vi "tx_top.vi"(0 "Modulation Parameters":T3 {"TX Parameters"."TX Sample Rate" items=["4M"]}) -> (9 "Transmitted IQ Graph":cluster{dbl[], dbl[]}(graph) caption="IQ Graph", 10 "Transmitted Magnitude":dbl[](graph), 11 "Transmitted Constellation Graph":T6(graph) caption="Constellation Graph", 13 "Transmitted Eye Diagram":cluster{"t0":dbl, "dt":dbl, "Y":dbl[]}[](graph) caption="Eye Diagram", 15 "Transmitted I":dbl[](graph), 16 "Transmitted Phase":dbl[](graph), 17 "Transmitted Q":dbl[](graph), 19 "Transmitted PSD":dbl[](graph), 20 "output IQ waveform":cluster{"t0":dbl, "dt":dbl, "Y":cdb[]}, 27 "error out":errorcluster)   [LabVIEW 2012]
uses:
  EE 497/LABS/SDR/control_type_defs.llb/tx_hw params.ctl
  EE 497/LABS/SDR/control_type_defs.llb/Queues.ctl
  gds_hw_config.lvlib
panel:
  in  "Queues in":T1
  in  "error in":errorcluster
  in  "STOP":bool
  out "Transmitting":bool
  out "Queues out":T1
  out "coerced gain (dB)":dbl format="%#_6f"
  out "coerced carrier frequency (Hz)":dbl format="%#_6p"
  out "data symbols":cdb[](array[numeric])=[0.0+0.0i, 0.7071067811865475+0.7071067811865475i, -0.7071067811865475-0.7071067811865475i, 0.7071067811865475-0.7071067811865475i, -0.7071067811865475-0.7071067811865475i, -0.7071067811865475+0.7071067811865475i, -0.7071067811865475+0.7071067811865475i, 0.7071067811865475-0.7071067811865475i, -0.7071067811865475+0.7071067811865475i, -0.7071067811865475-0.7071067811865475i, -0.7071067811865475+0.7071067811865475i, 0.7071067811865475-0.7071067811865475i, 0.7071067811865475+0.7071067811865475i, 0.7071067811865475-0.7071067811865475i, 0.7071067811865475-0.7071067811865475i, 0.7071067811865475+0.7071067811865475i, 0.7071067811865475+0.7071067811865475i, -0.7071067811865475+0.7071067811865475i, -0.7071067811865475+0.7071067811865475i, -0.7071067811865475-0.7071067811865475i, 0.7071067811865475-0.7071067811865475i, 0.7071067811865475+0.7071067811865475i, -0.7071067811865475-0.7071067811865475i, -0.7071067811865475-0.7071067811865475i, -0.7071067811865475-0.7071067811865475i, 0.7071067811865475-0.7071067811865475i, -0.7071067811865475+0.7071067811865475i, 0.7071067811865475-0.7071067811865475i, 0.7071067811865475+0.7071067811865475i, -0.7071067811865475+0.7071067811865475i, 0.7071067811865475-0.7071067811865475i, 0.7071067811865475-0.7071067811865475i, -0.7071067811865475+0.7071067811865475i, -0.7071067811865475-0.7071067811865475i, -0.7071067811865475-0.7071067811865475i, -0.7071067811865475-0.7071067811865475i, 0.7071067811865475+0.7071067811865475i, -0.7071067811865475+0.7071067811865475i, 0.7071067811865475-0.7071067811865475i, -0.7071067811865475+0.7071067811865475i, -0.7071067811865475+0.7071067811865475i, -0.7071067811865475+0.7071067811865475i, 0.7071067811865475-0.7071067811865475i, -0.7071067811865475+0.7071067811865475i, 0.7071067811865475-0.7071067811865475i, -0.7071067811865475+0.7071067811865475i, 0.7071067811865475+0.7071067811865475i, 0.7071067811865475+0.7071067811865475i, 0.7071067811865475+0.7071067811865475i, -0.7071067811865475-0.7071067811865475i, 0.7071067811865475+0.7071067811865475i, 0.7071067811865475-0.7071067811865475i, -0.7071067811865475+0.7071067811865475i, 0.7071067811865475-0.7071067811865475i, 0.7071067811865475-0.7071067811865475i, 0.7071067811865475+0.7071067811865475i, 0.7071067811865475-0.7071067811865475i, -0.7071067811865475+0.7071067811865475i, -0.7071067811865475+0.7071067811865475i, 0.7071067811865475-0.7071067811865475i, 0.7071067811865475-0.7071067811865475i, -0.7071067811865475-0.7071067811865475i, -0.7071067811865475-0.7071067811865475i, -0.7071067811865475-0.7071067811865475i, 0.7071067811865475-0.7071067811865475i, 0.7071067811865475+0.7071067811865475i, 0.7071067811865475-0.7071067811865475i, 0.7071067811865475-0.7071067811865475i, -0.7071067811865475+0.7071067811865475i, 0.7071067811865475+0.7071067811865475i, -0.7071067811865475-0.7071067811865475i, -0.7071067811865475+0.7071067811865475i, -0.7071067811865475+0.7071067811865475i, -0.7071067811865475-0.7071067811865475i, 0.7071067811865475+0.7071067811865475i, -0.7071067811865475+0.7071067811865475i, -0.7071067811865475-0.7071067811865475i, 0.7071067811865475+0.7071067811865475i, -0.7071067811865475-0.7071067811865475i, -0.7071067811865475-0.7071067811865475i, 0.7071067811865475+0.7071067811865475i, 0.7071067811865475-0.7071067811865475i, -0.7071067811865475-0.7071067811865475i, -0.7071067811865475-0.7071067811865475i, 0.7071067811865475-0.7071067811865475i, -0.7071067811865475-0.7071067811865475i, 0.7071067811865475-0.7071067811865475i, 0.7071067811865475+0.7071067811865475i, 0.7071067811865475+0.7071067811865475i, 0.7071067811865475-0.7071067811865475i, -0.7071067811865475+0.7071067811865475i, -0.7071067811865475+0.7071067811865475i, -0.7071067811865475-0.7071067811865475i, 0.7071067811865475-0.7071067811865475i, -0.7071067811865475+0.7071067811865475i, -0.7071067811865475-0.7071067811865475i, -0.7071067811865475+0.7071067811865475i, -0.7071067811865475-0.7071067811865475i, 0.7071067811865475+0.7071067811865475i, 0.7071067811865475+0.7071067811865475i, 0.7071067811865475-0.7071067811865475i, 0.7071067811865475-0.7071067811865475i, -0.7071067811865475+0.7071067811865475i, -0.7071067811865475+0.7071067811865475i, -0.7071067811865475-0.7071067811865475i, -0.7071067811865475-0.7071067811865475i, -0.7071067811865475+0.7071067811865475i, -0.7071067811865475+0.7071067811865475i, -0.7071067811865475+0.7071067811865475i, -0.7071067811865475+0.7071067811865475i, -0.7071067811865475+0.7071067811865475i, 0.7071067811865475+0.7071067811865475i, 0.7071067811865475+0.7071067811865475i, 0.7071067811865475-0.7071067811865475i, 0.7071067811865475-0.7071067811865475i, 0.7071067811865475+0.7071067811865475i, -0.7071067811865475+0.7071067811865475i, -0.7071067811865475+0.7071067811865475i, -0.7071067811865475-0.7071067811865475i, -0.7071067811865475-0.7071067811865475i, 0.7071067811865475+0.7071067811865475i, -0.7071067811865475+0.7071067811865475i, -0.7071067811865475-0.7071067811865475i, -0.7071067811865475+0.7071067811865475i, -0.7071067811865475-0.7071067811865475i, -0.7071067811865475+0.7071067811865475i, 0.7071067811865475+0.7071067811865475i, 0.7071067811865475+0.7071067811865475i, 0.7071067811865475-0.7071067811865475i, -0.7071067811865475-0.7071067811865475i, 0.7071067811865475+0.7071067811865475i, -0.7071067811865475-0.7071067811865475i, -0.7071067811865475+0.7071067811865475i, -0.7071067811865475+0.7071067811865475i, 0.7071067811865475-0.7071067811865475i, 0.7071067811865475+0.7071067811865475i, -0.7071067811865475-0.7071067811865475i, -0.7071067811865475-0.7071067811865475i, 0.7071067811865475-0.7071067811865475i, 0.7071067811865475-0.7071067811865475i, -0.7071067811865475-0.7071067811865475i, 0.7071067811865475-0.7071067811865475i, 0.7071067811865475-0.7071067811865475i, 0.7071067811865475+0.7071067811865475i, 0.7071067811865475-0.7071067811865475i, 0.7071067811865475+0.7071067811865475i, -0.7071067811865475+0.7071067811865475i, 0.7071067811865475+0.7071067811865475i, 0.7071067811865475-0.7071067811865475i, -0.7071067811865475+0.7071067811865475i, 0.7071067811865475-0.7071067811865475i, -0.7071067811865475-0.7071067811865475i, 0.7071067811865475+0.7071067811865475i, 0.7071067811865475+0.7071067811865475i, -0.7071067811865475+0.7071067811865475i, -0.7071067811865475-0.7071067811865475i, -0.7071067811865475-0.7071067811865475i, 0.7071067811865475-0.7071067811865475i, -0.7071067811865475+0.7071067811865475i, -0.7071067811865475-0.7071067811865475i, 0.7071067811865475+0.7071067811865475i, -0.7071067811865475-0.7071067811865475i, 0.7071067811865475-0.7071067811865475i, 0.7071067811865475+0.7071067811865475i, 0.7071067811865475+0.7071067811865475i, -0.7071067811865475-0.7071067811865475i, -0.7071067811865475+0.7071067811865475i, -0.7071067811865475-0.7071067811865475i, -0.7071067811865475-0.7071067811865475i, 0.7071067811865475+0.7071067811865475i, 0.7071067811865475+0.7071067811865475i, -0.7071067811865475-0.7071067811865475i, -0.7071067811865475-0.7071067811865475i, -0.7071067811865475-0.7071067811865475i, -0.7071067811865475-0.7071067811865475i, -0.7071067811865475+0.7071067811865475i, 0.7071067811865475+0.7071067811865475i, 0.7071067811865475+0.7071067811865475i, -0.7071067811865475-0.7071067811865475i, -0.7071067811865475-0.7071067811865475i, 0.7071067811865475-0.7071067811865475i, -0.7071067811865475-0.7071067811865475i, -0.7071067811865475-0.7071067811865475i, 0.7071067811865475+0.7071067811865475i, 0.7071067811865475-0.7071067811865475i, 0.7071067811865475-0.7071067811865475i, -0.7071067811865475-0.7071067811865475i, 0.7071067811865475+0.7071067811865475i, -0.7071067811865475-0.7071067811865475i, 0.7071067811865475+0.7071067811865475i, -0.7071067811865475+0.7071067811865475i, 0.7071067811865475+0.7071067811865475i, 0.7071067811865475+0.7071067811865475i, -0.7071067811865475+0.7071067811865475i, 0.7071067811865475-0.7071067811865475i, 0.7071067811865475-0.7071067811865475i, 0.7071067811865475+0.7071067811865475i, -0.7071067811865475-0.7071067811865475i, -0.7071067811865475+0.7071067811865475i, -0.7071067811865475-0.7071067811865475i, 0.7071067811865475-0.7071067811865475i, 0.7071067811865475+0.7071067811865475i, 0.7071067811865475-0.7071067811865475i, -0.7071067811865475-0.7071067811865475i, -0.7071067811865475+0.7071067811865475i, 0.7071067811865475-0.7071067811865475i, -0.7071067811865475-0.7071067811865475i, -0.7071067811865475-0.7071067811865475i, 0.7071067811865475+0.7071067811865475i, -0.7071067811865475-0.7071067811865475i, 0.7071067811865475-0.7071067811865475i, -0.7071067811865475+0.7071067811865475i, 0.7071067811865475+0.7071067811865475i, -0.7071067811865475+0.7071067811865475i, -0.7071067811865475+0.7071067811865475i, -0.7071067811865475+0.7071067811865475i, 0.7071067811865475-0.7071067811865475i, 0.7071067811865475+0.7071067811865475i, 0.7071067811865475-0.7071067811865475i, -0.7071067811865475-0.7071067811865475i, 0.7071067811865475+0.7071067811865475i, 0.7071067811865475-0.7071067811865475i, -0.7071067811865475+0.7071067811865475i, -0.7071067811865475-0.7071067811865475i, 0.7071067811865475-0.7071067811865475i, 0.7071067811865475-0.7071067811865475i, 0.7071067811865475-0.7071067811865475i, -0.7071067811865475-0.7071067811865475i, 0.7071067811865475+0.7071067811865475i, 0.7071067811865475-0.7071067811865475i, 0.7071067811865475+0.7071067811865475i, -0.7071067811865475-0.7071067811865475i, 0.7071067811865475+0.7071067811865475i, 0.7071067811865475-0.7071067811865475i, 0.7071067811865475+0.7071067811865475i, 0.7071067811865475-0.7071067811865475i, 0.7071067811865475+0.7071067811865475i, 0.7071067811865475+0.7071067811865475i, 0.7071067811865475+0.7071067811865475i, 0.7071067811865475+0.7071067811865475i, -0.7071067811865475+0.7071067811865475i, 0.7071067811865475+0.7071067811865475i, 0.7071067811865475-0.7071067811865475i, 0.7071067811865475+0.7071067811865475i, 0.7071067811865475-0.7071067811865475i, -0.7071067811865475+0.7071067811865475i, 0.7071067811865475+0.7071067811865475i, 0.7071067811865475-0.7071067811865475i, 0.7071067811865475+0.7071067811865475i, -0.7071067811865475-0.7071067811865475i]
  out "key bit sequence":u8[](array[numeric])=[0, 0, 0, 0, 0, 0, 0, 0, 1, 1, 1, 0, 1, 0, 0, 1, 1, 0, 1, 1, 1, 0, 0, 1, 0, 0, 0, 1, 0, 1, 0, 0, 0, 0, 1, 0, 1, 0, 1, 1, 0, 1, 0, 0, 1, 1, 1, 1, 1, 1, 0, 1, 1, 0, 0, 1, 0, 0, 1, 0, 0, 1, 0, 1, 1, 0, 1, 1, 1, 1, 1, 1, 0, 0, 1, 0, 0, 1, 1, 0, 1, 0, 1, 0, 0, 1, 1, 0, 0, 1, 1, 0, 0, 0, 0, 0, 0, 0, 1, 1, 0, 0, 0, 1, 1, 0, 0, 1, 0, 1, 0, 0, 0, 1, 1, 0, 1, 0, 0, 1, 0, 1, 1, 1, 1, 1, 1, 1, 0, 1, 0, 0, 0, 1, 0, 1, 1, 0, 0, 0, 1, 1, 1, 0, 1, 0, 1, 1, 0, 0, 1, 0, 1, 1, 0, 0, 1, 1, 1, 1, 0, 0, 0, 1, 1, 1, 1, 1, 0, 1, 1, 1, 0, 1, 0, 0, 0, 0, 0, 1, 1, 0, 1, 0, 1, 1, 0, 1, 1, 0, 1, 1, 1, 0, 1, 1, 0, 0, 0, 0, 0, 1, 0, 1, 1, 0, 1, 0, 1, 1, 1, 1, 1, 0, 1, 0, 1, 0, 1, 0, 1, 0, 0, 0, 0, 0, 0, 1, 0, 1, 0, 0, 1, 0, 1, 0, 1, 1, 1, 1, 0, 0, 1, 0, 1, 1, 1, 0, 1, 1, 1, 0, 0, 0, 0, 0, 0, 1, 1, 1, 0, 0, 1, 1, 1, 0, 1, 0, 0, 1, 0, 0, 1, 1, 1, 1, 0, 1, 0, 1, 1, 1, 0, 1, 0, 1, 0, 0, 0, 1, 0, 0, 1, 0, 0, 0, 0, 1, 1, 0, 0, 1, 1, 1, 0, 0, 0, 0, 1, 0, 1, 1, 1, 1, 0, 1, 1, 0, 1, 1, 0, 0, 1, 1, 0, 1, 0, 0, 0, 0, 1, 1, 1, 0, 1, 1, 1, 1, 0, 0, 0, 0, 1, 1, 1, 1, 1, 1, 1, 1, 1, 0, 0, 0, 0, 0, 1, 1, 1, 1, 0, 1, 1, 1, 1, 1, 0, 0, 0, 1, 0, 1, 1, 1, 0, 0, 1, 1, 0, 0, 1, 0, 0, 0, 0, 0, 1, 0, 0, 1, 0, 1, 0, 0, 1, 1, 1, 0, 1, 1, 0, 1, 0, 0, 0, 1, 1, 1, 1, 0, 0, 1, 1, 1, 1, 1, 0, 0, 1, 1, 0, 1, 1, 0, 0, 0, 1, 0, 1, 0, 1, 0, 0, 1, 0, 0, 0, 1, 1, 1, 0, 0, 0, 1, 1, 0, 1, 1, 0, 1, 0, 1, 0, 1, 1, 1, 0, 0, 0, 1, 0, 0, 1, 1, 0, 0, 0, 1, 0, 0, 0, 1, 0, 0, 0, 0, 0, 0, 0, 0, 1, 0, 0, 0, 0, 1, 0, 0, 0, 1, 1, 0, 0, 0, 0, 1, 0, 0, 1, 1]
  out "packet duration (sec)":dbl min=50000000.0 max=100000000.0 step=50000000.0 format="%#_6p"
  out "symbol rate (Hz)":dbl min=50000000.0 max=100000000.0 step=50000000.0 format="%#_6p"
  in  "Configurations":T2(tab)
  in  "HW parameters":T4={"Device IP Address"="192.168.11.3", "Active Antenna"="TX1", "Carrier Frequency (Hz)"=915000000.0, "Gain (dB)"=10.0, "Generation Mode"=enum."continuous"} {"Gain (dB)" format="%.2f"; "Carrier Frequency (Hz)" format="%.2p"}
  in  "TX Graphs":T5(tab)
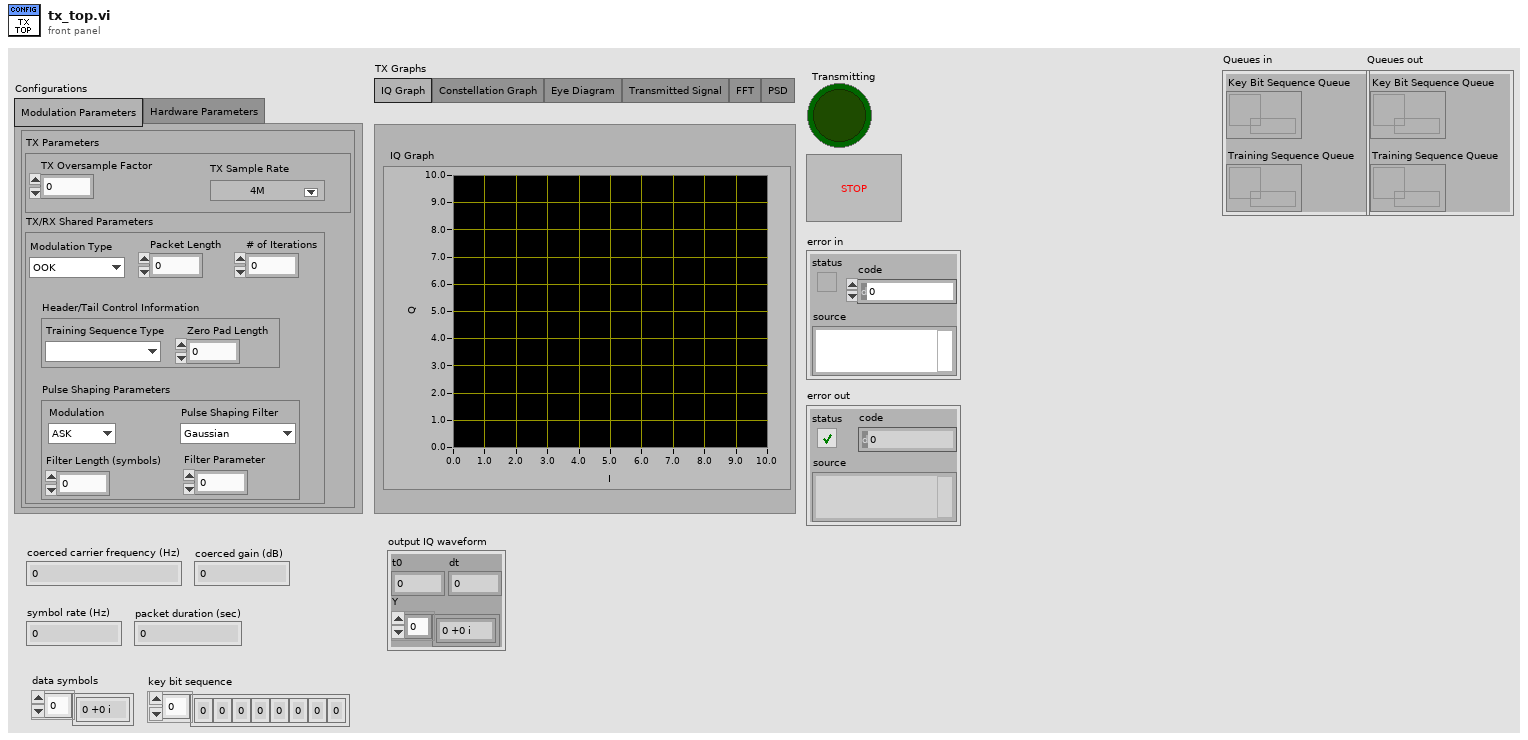
[diagram p1: front panel]
types:
  T1 = typedef "Queues.ctl" = cluster{"Key Bit Sequence Queue":refnum<queue>, "Training Sequence Queue":refnum<queue>}
  T2 = enum32{"Modulation Parameters", "Hardware Parameters"}
  T3 = cluster{"TX Parameters":cluster{"TX Oversample Factor":u16, "TX Sample Rate":dbl}, "TX/RX Shared Parameters":cluster{"Modulation Type":enum16{"OOK", "FSK"}, "Packet Length":dbl, "# of Iterations":dbl, "Pulse Shaping Parameters":cluster{"Modulation":enum16{"ASK", "FSK", "PSK", "QAM", "MSK", "PAM"}, "Pulse Shaping Filter":enum16{"Gaussian"}, "Filter Length (symbols)":dbl, "Filter Parameter":dbl}, "Header/Tail Control Information":cluster{"Training Sequence Type":enum16{""}, "Zero Pad Length":dbl}}}
  T4 = typedef "tx_hw params.ctl" = cluster{"Device IP Address":refnum<k15>, "Active Antenna":string, "Carrier Frequency (Hz)":dbl, "Gain (dB)":dbl, "Generation Mode":enum16{"single shot", "simulate", "continuous"}}
  T5 = enum32{"IQ Graph", "Constellation Graph", "Eye Diagram", "Transmitted Signal", "FFT", "PSD"}
  T6 = cluster{"Decimated Array":dbl[], "Decimated Array":dbl[]}[]
  T7 = cluster{"TX Parameters":cluster{"TX Oversample Factor":dbl, "TX Sample Rate":dbl}, "TX/RX Shared Parameters":cluster{"Modulation Type":enum16{"OOK", "FSK"}, "Packet Length":dbl, "# of Iterations":dbl, "Pulse Shaping Parameters":cluster{"Modulation":enum16{"ASK", "FSK", "PSK", "QAM", "MSK", "PAM"}, "Pulse Shaping Filter":enum16{"Gaussian"}, "Filter Length (symbols)":dbl, "Filter Parameter":dbl}, "Header/Tail Control Information":cluster{"Training Sequence Type":enum16{""}, "Zero Pad Length":dbl}}}
  T8 = cluster{"TX Oversample Factor":u16, "TX Sample Rate":dbl}
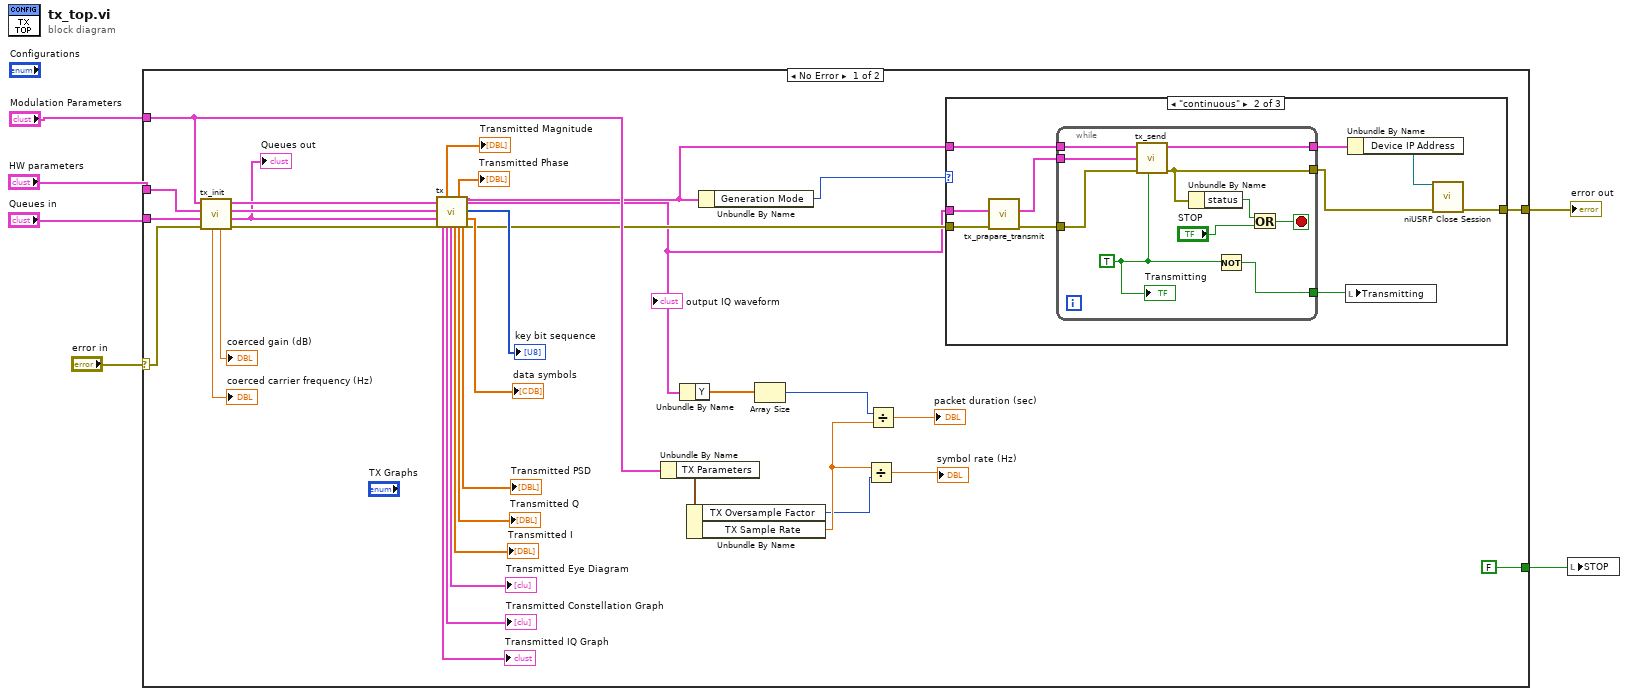
[diagram p0: block diagram]
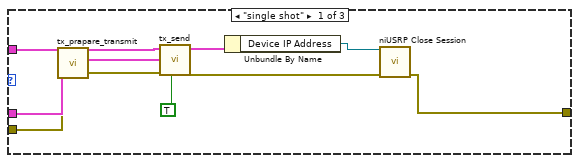
[diagram p2: hidden frame]
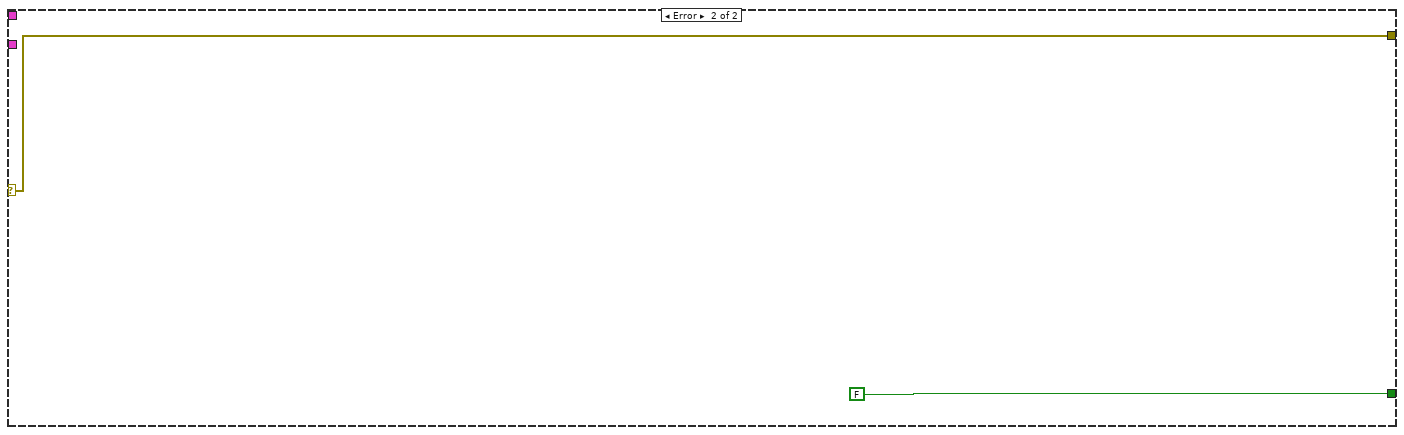
[diagram p4: hidden frame]
diagram:
  n1 = case shown="No Error" "error in" {
    selector: "error in" -> [w37 w71]
    tunnel: "HW parameters" -> [w36 _]
    tunnel: "Modulation Parameters" -> [w24 _]
    tunnel: "Queues in" -> [w35 _]
    tunnel: [FALSE FALSE ("Done")] -> w2
    tunnel: [w10 w71] -> w1
    frame No Error {
      n2 = call "tx_init.vi"("error in (no error)"=w37, "Queues in"=w35, "HW parameters In"=w36, "Modulation Parameters In"=w24) -> ("error out"=w34:errorcluster, "Queues out"=w9:T1, "HW parameters out"=w13:T4, "Modulation Parameters Out"=w12:T7, "coerced gain (dB)"=→"coerced gain (dB)":dbl, "coerced carrier frequency (Hz)"=→"coerced carrier frequency (Hz)":dbl)  [unwired: 2 in]
      "Queues out" <- w9
      n3 = call "tx.vi"("Modulation Parameters In"=w12, "HW parameters in"=w13, "Queues in"=w9, "error in"=w34) -> ("Transmitted IQ Graph"=→"Transmitted IQ Graph":cluster{dbl[], dbl[]}, "Transmitted Magnitude"=→"Transmitted Magnitude":dbl[], "Transmitted Constellation Graph"=→"Transmitted Constellation Graph":T6, "Transmitted Eye Diagram"=→"Transmitted Eye Diagram":cluster{"t0":dbl, "dt":dbl, "Y":dbl[]}[], "Transmitted I"=→"Transmitted I":dbl[], "Transmitted Phase"=→"Transmitted Phase":dbl[], "Transmitted Q"=→"Transmitted Q":dbl[], "Transmitted PSD"=→"Transmitted PSD":dbl[], "HW parameters out"=w7:T4, "output complex waveform"=w8:cluster{"t0":dbl, "dt":dbl, "Y":cdb[]}, "key bit sequence"=→"key bit sequence":u8[], "data symbols"=→"data symbols":cdb[], "error out"=w11:errorcluster)  [unwired: 11 in]
      "output IQ waveform" <- w8
      n4 = Unbundle By Name(w24) -> ("TX Parameters"=w25:T8)
      n5 = Unbundle By Name(w8) -> ("Y"=w23:cdb[])
      n6 = Unbundle By Name(w25) -> ("TX Oversample Factor"=w20:u16, "TX Sample Rate"=w21:dbl)
      n7 = Unbundle By Name(w7) -> ("Generation Mode"=w16:enum16{"single shot", "simulate", "continuous"})
      n8 = Array Size(array=w23) -> (size(s)=w22:i32)
      n9 = Divide(x=w21, y=w20) -> (x/y=→"symbol rate (Hz)":dbl)
      n10 = Divide(x=w22, y=w21) -> (x/y=→"packet duration (sec)":dbl)
      n11 = case shown="\"continuous\"" w16 {
        tunnel: w8 -> [w49 w59 _]
        tunnel: w11 -> [w48 w58 w70]
        tunnel: [w47 w54 w70] -> w10
        tunnel: w7 -> [w43 w52 _]
        frame "single shot" {
          n12 = call "tx_prapare_transmit.vi"("error in (no error)"=w48, "input IQ waveform"=w49) -> ("error out"=w45:errorcluster, "Scaled and Padded IQ waveform"=w44:cluster{"t0":dbl, "dt":dbl, "Y":cdb[]})  [unwired: 8 in]
          n13 = call "tx_send.vi"("end of data?"=TRUE, "error in (no error)"=w45, "IQ Data in"=w44, "HW parameters in"=w43) -> ("error out"=w46:errorcluster, "HW parameters out"=w42:T4)  [unwired: 6 in]
          n14 = Unbundle By Name(w42) -> ("Device IP Address"=w41:refnum<k15>)
          n15 = call <instrlib>:"niUSRP Close Session.vi"("session handle"=w41, "error in (no error)"=w46) -> ("error out"=w47:errorcluster)  [unwired: 13 in]
        }
        frame "continuous" {
          n16 = call "tx_prapare_transmit.vi"("error in (no error)"=w58, "input IQ waveform"=w59) -> ("error out"=w57:errorcluster, "Scaled and Padded IQ waveform"=w53:cluster{"t0":dbl, "dt":dbl, "Y":cdb[]})  [unwired: 8 in]
          n17 = while {
            tunnel: w57 -> [w69]
            tunnel: [w65] -> w56
            tunnel: [w64] -> w55
            tunnel: w53 -> [w62]
            tunnel: w52 -> [w61]
            tunnel: [w60] -> w51
            stop <- w66 stop-if-true
            w63 = TRUE
            n18 = call "tx_send.vi"("end of data?"=w63, "error in (no error)"=w69, "IQ Data in"=w62, "HW parameters in"=w61) -> ("error out"=w64:errorcluster, "HW parameters out"=w60:T4)  [unwired: 6 in]
            n19 = Unbundle By Name(w64) -> ("status"=w68:bool)
            n20 = Not(x=w63) -> (.not. x?=w65:bool)
            n21 = Or(x=w68, y="STOP") -> (x .or. y?=w66:bool)
            "Transmitting" <- w63
          }
          n22 = local write "Transmitting"(w56) -> ()
          n23 = Unbundle By Name(w51) -> ("Device IP Address"=w50:refnum<k15>)
          n24 = call <instrlib>:"niUSRP Close Session.vi"("session handle"=w50, "error in (no error)"=w55) -> ("error out"=w54:errorcluster)  [unwired: 13 in]
        }
        frame "simulate", Default {
        }
      }
    }
    frame Error {
    }
  }
  "error out" <- w1
  n25 = local write "STOP"(w2) -> ()
